vi "seti_labview_read_parameters_from_file.vi"(8 "error in (no error)":errorcluster, 11 "Run Number\nto Load":i32=1) -> (0 "error out":errorcluster, 1 "start_icfft":i32, 2 "Chirp FFT Pairs":T2[](array[typedef]), 3 "binWorkUnitDataPoints.bin (DataIn)":csg[](array[numeric]), 4 "Array of Power Spectrum Data":T1[](array[typedef]), 5 "NumDataPoints":u32, 7 "end_icfft":i32)   [LabVIEW 2015, in "SETI_LV.lvlib"]
uses:
  SETI_LV.lvlib
  TypeDefs/ChirpFFT Pairs.ctl
  TypeDefs/Power Spectrum Data.ctl
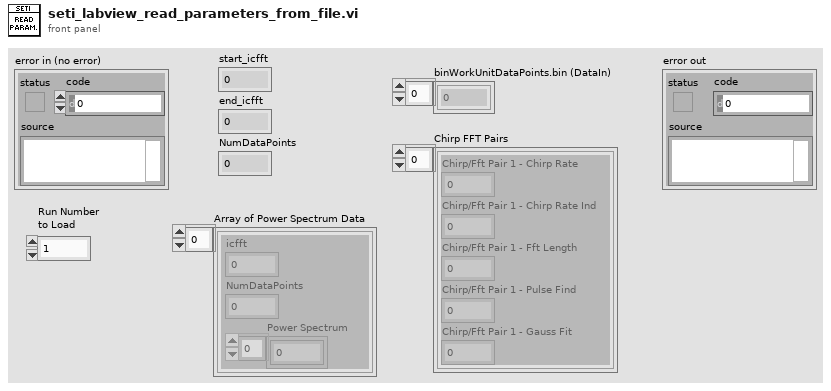
[diagram p1: front panel]
types:
  T1 = typedef "SETI_LV.lvlib/Power Spectrum Data.ctl" = cluster{"icfft":i32, "NumDataPoints":i32, "Power Spectrum":sgl[]}
  T2 = typedef "SETI_LV.lvlib/ChirpFFT Pairs.ctl" = cluster{"Chirp/Fft Pair 1 - Chirp Rate":dbl, "Chirp/Fft Pair 1 - Chirp Rate Ind":i32, "Chirp/Fft Pair 1 - Fft Length":i32, "Chirp/Fft Pair 1 - Pulse Find":i32, "Chirp/Fft Pair 1 - Gauss Fit":i32}
  T3 = enum16{"big-endian, network order", "native, host order", "little-endian"}
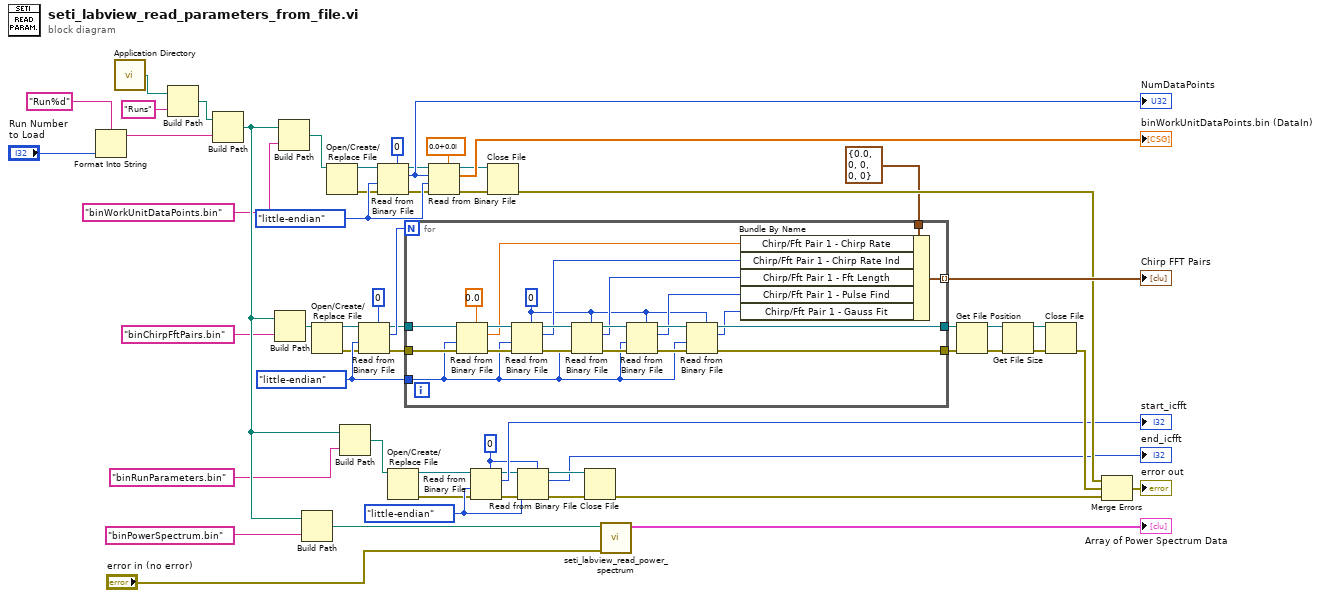
[diagram p0: block diagram]
diagram:
  w34 = T3."little-endian" ("byte order (0:big-endian, network order)")
  w40 = 0
  w19 = T3."little-endian" ("byte order (0:big-endian, network order)")
  w39 = T3."little-endian" ("byte order (0:big-endian, network order)")
  n1 = Format Into String(format string="Run%d", "Run Number\nto Load") -> (resulting string=w1:string)  [unwired: 2 in, 1 out]
  n2 = call <vilib>:"Application Directory.vi"() -> ("Application Directory"=w3:path)
  n3 = Build Path(base path=w3, name or relative path="Runs") -> (appended path=w47:path)
  n4 = Build Path(base path=w47, name or relative path=w1) -> (appended path=w48:path)
  n5 = Build Path(base path=w48, name or relative path="binChirpFftPairs.bin") -> (appended path=w12:path)
  n6 = Build Path(base path=w48, name or relative path="binWorkUnitDataPoints.bin") -> (appended path=w10:path)
  n7 = Build Path(base path=w48, name or relative path="binPowerSpectrum.bin") -> (appended path=w43:path)
  n8 = Open/Create/Replace File(file path (use dialog)=w12) -> (refnum out=w17:refnum<file>, error out=w16:errorcluster)  [unwired: 5 in, 1 out]
  n9 = Open/Create/Replace File(file path (use dialog)=w10) -> (refnum out=w4:refnum<file>, error out=w5:errorcluster)  [unwired: 5 in, 1 out]
  n10 = Build Path(base path=w48, name or relative path="binRunParameters.bin") -> (appended path=w31:path)
  n11 = Read from Binary File(5:0, 8:w16, 9:w19, 11:w17) -> (0:w18:errorcluster, 2:w20:i32, 3:w14:refnum<file>)  [unwired: 2 in, 1 out]
  n12 = Read from Binary File(5:u32 0, 8:w5, 9:w39, 11:w4) -> (0:w37:errorcluster, 2:w44:u32, 3:w8:refnum<file>)  [unwired: 2 in, 1 out]
  "NumDataPoints" <- w44
  n13 = Open/Create/Replace File(file path (use dialog)=w31) -> (refnum out=w28:refnum<file>, error out=w29:errorcluster)  [unwired: 5 in, 1 out]
  n14 = for {
    N: w20 -> [_]
    tunnel: w14 -> [w78]
    tunnel: w18 -> [w77]
    tunnel: w19 -> [w68]
    tunnel: [w67] -> w22
    tunnel: [w66] -> w23
    tunnel: T2 {"Chirp/Fft Pair 1 - Chirp Rate"=0.0, "Chirp/Fft Pair 1 - Chirp Rate Ind"=0, "Chirp/Fft Pair 1 - Fft Length"=0, "Chirp/Fft Pair 1 - Pulse Find"=0, "Chirp/Fft Pair 1 - Gauss Fit"=0} ("Chirp/Fft Pairs") -> [w65]
    tunnel: [w59] -> w54 mode=indexing
    w58 = 0
    n15 = Read from Binary File(5:0.0, 8:w77, 9:w68, 11:w78) -> (0:w75:errorcluster, 2:w64:dbl, 3:w76:refnum<file>)  [unwired: 2 in, 1 out]
    n16 = Read from Binary File(5:w58, 8:w75, 9:w68, 11:w76) -> (0:w73:errorcluster, 2:w63:i32, 3:w74:refnum<file>)  [unwired: 2 in, 1 out]
    n17 = Read from Binary File(5:w58, 8:w73, 9:w68, 11:w74) -> (0:w69:errorcluster, 2:w62:i32, 3:w70:refnum<file>)  [unwired: 2 in, 1 out]
    n18 = Read from Binary File(5:w58, 8:w69, 9:w68, 11:w70) -> (0:w72:errorcluster, 2:w61:i32, 3:w71:refnum<file>)  [unwired: 2 in, 1 out]
    n19 = Read from Binary File(5:w58, 8:w72, 9:w68, 11:w71) -> (0:w66:errorcluster, 2:w60:i32, 3:w67:refnum<file>)  [unwired: 2 in, 1 out]
    n20 = Bundle By Name(cluster=w65, "Chirp/Fft Pair 1 - Chirp Rate"=w64, "Chirp/Fft Pair 1 - Chirp Rate Ind"=w63, "Chirp/Fft Pair 1 - Fft Length"=w62, "Chirp/Fft Pair 1 - Pulse Find"=w61, "Chirp/Fft Pair 1 - Gauss Fit"=w60) -> (w59:T2)
  }
  "Chirp FFT Pairs" <- w54
  n21 = Read from Binary File(5:csg 0.0+0.0i, 8:w37, 9:w39, 10:w44, 11:w8) -> (0:w38:errorcluster, 2:→"binWorkUnitDataPoints.bin (DataIn)":csg[], 3:w7:refnum<file>)  [unwired: 1 in, 1 out]
  n22 = Read from Binary File(5:w40, 8:w29, 9:w34, 11:w28) -> (0:w33:errorcluster, 2:→"start_icfft":i32, 3:w32:refnum<file>)  [unwired: 2 in, 1 out]
  n23 = Close File(refnum=w7, error in=w38) -> (error out=w51:errorcluster)  [unwired: 1 out]
  n24 = Read from Binary File(5:w40, 8:w33, 9:w34, 11:w32) -> (0:w36:errorcluster, 2:→"end_icfft":i32, 3:w35:refnum<file>)  [unwired: 2 in, 1 out]
  n25 = Close File(refnum=w35, error in=w36) -> (error out=w49:errorcluster)  [unwired: 1 out]
  n26 = call "seti_labview_read_power_spectrum.vi"("error in (no error)"="error in (no error)", "Power Spectrum Data file path"=w43) -> ("Array of Power Spectrum Data"=→"Array of Power Spectrum Data":T1[])  [unwired: 8 in, 1 out]
  n27 = Get File Position(4:w23, 7:w22) -> (0:w24:errorcluster, 3:w25:refnum<file>)  [unwired: 1 out]
  n28 = Get File Size(file=w25, error in=w24) -> (refnum out=w26:refnum<file>, 0:w27:errorcluster)  [unwired: 1 out]
  n29 = Close File(refnum=w26, error in=w27) -> (error out=w50:errorcluster)  [unwired: 1 out]
  n30 = Merge Errors(w51, w50, w49) -> (→"error out":errorcluster)
